vi "Reorder cluster elements.vi"(8 "error in (no error)":errorcluster, 10 "Reference Variant":variant, 11 "Data Variant":variant) -> (0 "error out":errorcluster, 1 "Reference key names":string[](array[string]), 2 "Ordered VCluster":variant, 3 "Queried key names":string[](array[string]), 4 "Current element name":string)   [LabVIEW 2015]
uses:
  <vilib>/Utility/Data Type/NI_Data Type.lvlib
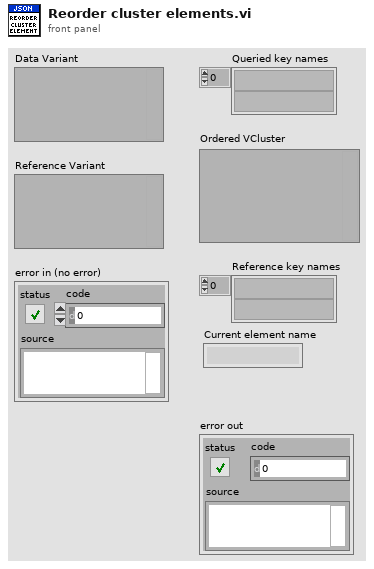
[diagram p1: front panel]
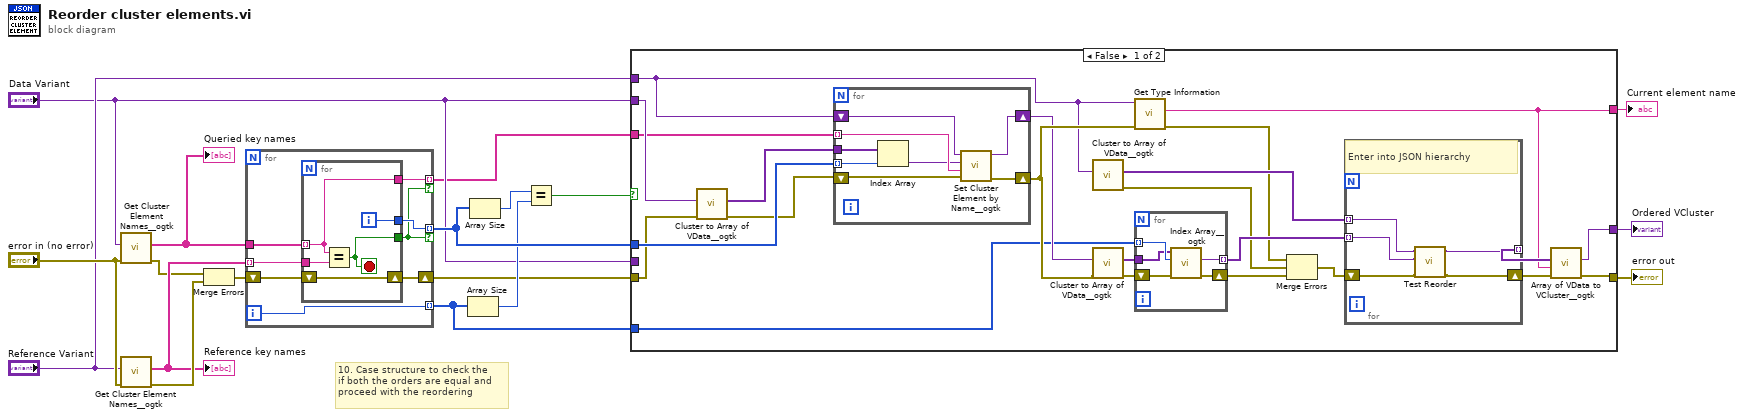
[diagram p0: block diagram]
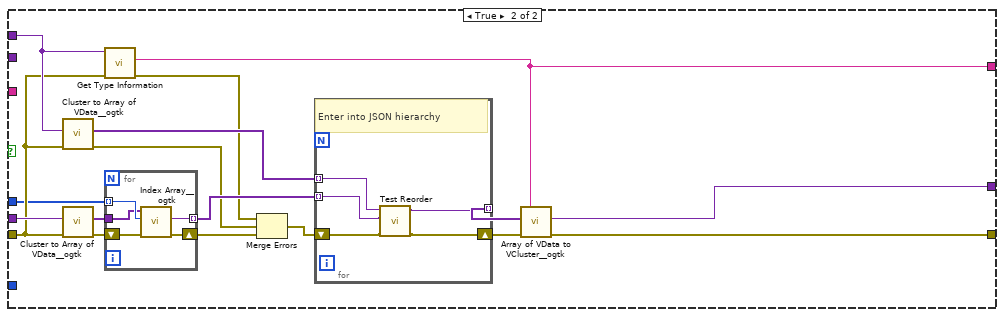
[diagram p2: hidden frame]
diagram:
  # "10. Case structure to check the\nif both the orders are equal and \nproceed with the reordering"
  n1 = call <userlib>:"Get Cluster Element Names__ogtk.vi"("error in (no error)"="error in (no error)", "Cluster"="Data Variant") -> ("error out"=w11:errorcluster, "Element Names"=w16:string[])  [unwired: 8 in]
  "Queried key names" <- w16
  n2 = call <userlib>:"Get Cluster Element Names__ogtk.vi"("error in (no error)"="error in (no error)", "Cluster"="Reference Variant") -> ("error out"=w17:errorcluster, "Element Names"=w15:string[])  [unwired: 8 in]
  "Reference key names" <- w15
  n3 = Merge Errors(w11, w17) -> (w18:errorcluster)
  n4 = for {
    tunnel: w15 -> [w25] mode=indexing
    tunnel: w16 -> [w26]
    tunnel: [w24] -> w9 mode=indexing if=w19
    shift-right: [w22] -> w3
    shift-left: w18 -> [w23]
    tunnel: [w21] -> w2 mode=indexing
    tunnel: [w20] -> w4 mode=indexing if=w19
    i -> [w21]
    n5 = for {
      tunnel: w26 -> [w27] mode=indexing
      tunnel: w25 -> [w31]
      tunnel: [w30] -> w24
      shift-right: [w29] -> w22
      shift-left: w23 -> [w29]
      tunnel: [w28] -> w19
      tunnel: [w27] -> w20
      i -> [w30]
      stop <- w28 stop-if-true
      n6 = Equal?(x=w27, y=w31) -> (x = y?=w28:bool)
    }
  }
  n7 = Array Size(array=w2) -> (size(s)=w7:i32)
  n8 = Array Size(array=w9) -> (size(s)=w8:i32)
  n9 = Equal?(x=w8, y=w7) -> (x = y?=w6:bool)
  n10 = case shown="False" w6 {
    tunnel: w9 -> [w52 w74]
    tunnel: w3 -> [w49 w75]
    tunnel: "Reference Variant" -> [w36 w83]
    tunnel: "Data Variant" -> [_ w87]
    tunnel: [w38 w79] -> w12
    tunnel: [w35 w85] -> w10
    tunnel: "Data Variant" -> [w54 _]
    tunnel: w4 -> [w51 _]
    tunnel: w2 -> [w33 _]
    tunnel: [w32 w73] -> w1
    frame False {
      n11 = call <userlib>:"Cluster to Array of VData__ogtk.vi"("error in (no error)"=w49, "Cluster"=w54) -> ("error out"=w50:errorcluster, "Array of VData"=w53:variant[])  [unwired: 8 in]
      n12 = for {
        tunnel: w53 -> [w72]
        tunnel: w52 -> [w65] mode=indexing
        tunnel: w51 -> [w71] mode=indexing
        shift-right: [w67] -> w37
        shift-left: w50 -> [w68]
        shift-right: [w66] -> w34
        shift-left: w36 -> [w70]
        n13 = Index Array(array=w72, index=w65) -> (element=w69:variant)
        n14 = call <userlib>:"Set Cluster Element by Name__ogtk.vi"("error in (no error)"=w68, "Element Name (\"\": New Element Data Name)"=w71, "New Element Value"=w69, "Cluster"=w70) -> ("error out"=w67:errorcluster, "VCluster out"=w66:variant)  [unwired: 5 in, 1 out]
      }
      n15 = call <userlib>:"Cluster to Array of VData__ogtk.vi"("Cluster"=w36) -> ("error out"=w40:errorcluster, "Array of VData"=w44:variant[])  [unwired: 9 in]
      n16 = call <userlib>:"Cluster to Array of VData__ogtk.vi"("error in (no error)"=w37, "Cluster"=w34) -> ("error out"=w48:errorcluster, "Array of VData"=w47:variant[])  [unwired: 8 in]
      n17 = call <vilib>:"Get Type Information.vi"("error in (no error)"=w37, "Variant"=w36) -> ("error out"=w39:errorcluster, "Name"=w32:string)  [unwired: 5 in, 3 out]
      n18 = for {
        tunnel: w47 -> [w60]
        shift-right: [w61] -> w46
        shift-left: w48 -> [w62]
        tunnel: w33 -> [w64] mode=indexing
        tunnel: [w63] -> w45 mode=indexing
        n19 = call <userlib>:"Index Array__ogtk.vi"("error in (no error)"=w62, "Index (1D)"=w64, "MultiD Array"=w60) -> ("error out"=w61:errorcluster, "Array Element"=w63:variant)  [unwired: 7 in]
      }
      n20 = Merge Errors(w39, w40, w46) -> (w43:errorcluster)
      n21 = for {
        shift-right: [w55] -> w42
        shift-left: w43 -> [w59]
        tunnel: w45 -> [w57] mode=indexing
        tunnel: w44 -> [w58] mode=indexing
        tunnel: [w56] -> w41 mode=indexing
        # "Enter into JSON hierarchy"
        n22 = call "Test Reorder.vi"("error in (no error)"=w59, "Data Variant"=w57, "Reference Variant"=w58) -> ("error out"=w55:errorcluster, "Output VData"=w56:variant)  [unwired: 6 in, 1 out]
      }
      n23 = call <userlib>:"Array of VData to VCluster__ogtk.vi"("error in (no error)"=w42, "Cluster Name"=w32, "Array"=w41) -> ("error out"=w38:errorcluster, "VCluster"=w35:variant)  [unwired: 7 in]
    }
    frame True {
      n24 = call <userlib>:"Cluster to Array of VData__ogtk.vi"("error in (no error)"=w75, "Cluster"=w83) -> ("error out"=w77:errorcluster, "Array of VData"=w82:variant[])  [unwired: 8 in]
      n25 = call <userlib>:"Cluster to Array of VData__ogtk.vi"("error in (no error)"=w75, "Cluster"=w87) -> ("error out"=w89:errorcluster, "Array of VData"=w88:variant[])  [unwired: 8 in]
      n26 = call <vilib>:"Get Type Information.vi"("error in (no error)"=w75, "Variant"=w83) -> ("error out"=w76:errorcluster, "Name"=w73:string)  [unwired: 5 in, 3 out]
      n27 = for {
        tunnel: w88 -> [w95]
        shift-right: [w96] -> w86
        shift-left: w89 -> [w97]
        tunnel: w74 -> [w99] mode=indexing
        tunnel: [w98] -> w84 mode=indexing
        n28 = call <userlib>:"Index Array__ogtk.vi"("error in (no error)"=w97, "Index (1D)"=w99, "MultiD Array"=w95) -> ("error out"=w96:errorcluster, "Array Element"=w98:variant)  [unwired: 7 in]
      }
      n29 = Merge Errors(w76, w77, w86) -> (w81:errorcluster)
      n30 = for {
        shift-right: [w93] -> w80
        shift-left: w81 -> [w94]
        tunnel: w84 -> [w91] mode=indexing
        tunnel: w82 -> [w92] mode=indexing
        tunnel: [w90] -> w78 mode=indexing
        # "Enter into JSON hierarchy"
        n31 = call "Test Reorder.vi"("error in (no error)"=w94, "Data Variant"=w91, "Reference Variant"=w92) -> ("error out"=w93:errorcluster, "Output VData"=w90:variant)  [unwired: 6 in, 1 out]
      }
      n32 = call <userlib>:"Array of VData to VCluster__ogtk.vi"("error in (no error)"=w80, "Cluster Name"=w73, "Array"=w78) -> ("error out"=w79:errorcluster, "VCluster"=w85:variant)  [unwired: 7 in]
    }
  }
  "error out" <- w12
  "Ordered VCluster" <- w10
  "Current element name" <- w1
